vi "test_rethinkdb_reql_encode.vi"() -> ()   [LabVIEW 2017]
uses:
  rethinkdb/rethinkdb.lvlib
panel:
  out "reql":string
  out "error out":errorcluster
  in  "Cluster":T1={"Boolean"=TRUE, "int"=-123, "float"=3.14, "String"="hello\nworld", "Array"=[1, 2, 3], "Objects"=[{"SubArray"=["a", "b"], "Boolean"=TRUE}, {"SubArray"=[], "Boolean"=FALSE}]}
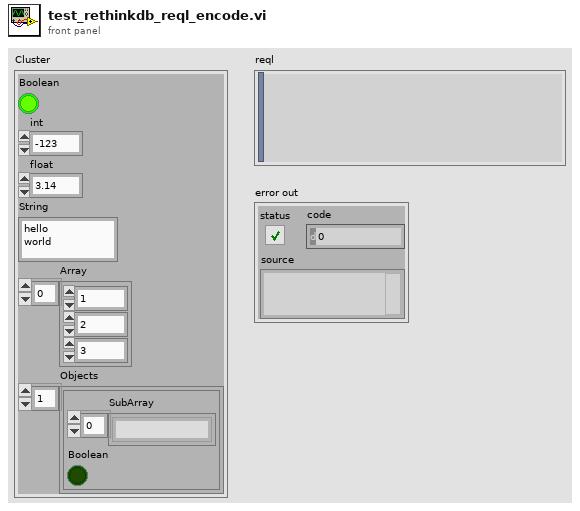
[diagram p1: front panel]
types:
  T1 = cluster{"Boolean":bool, "int":i32, "float":dbl, "String":string, "Array":u8[], "Objects":cluster{"SubArray":string[], "Boolean":bool}[]}
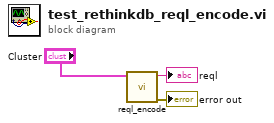
[diagram p0: block diagram]
diagram:
  n1 = call "reql_encode.vi"("object"="Cluster") -> ("error out"=→"error out":errorcluster, "reql"=→"reql":string)  [unwired: 9 in]
